vi "lockin - Set REF phase equals zero.vi"(9 "reset REF phi to zero":bool, 10 "Channels: Lockin":T1={"REF f (Hz)"=[0.4, 0.4], "REF phi (deg)"=[0.0, 0.0]} {"REF phi (deg)" format="%#_3g"}, 11 "Channels: AO":T2={"AO amp (V)"=[0.0, 0.0, 0.0, 0.0, 0.0, 0.0, 0.0, 0.0], "AO DC (V)"=[0.0, 0.0, 0.0, 0.0, 0.0, 0.0, 0.0, 0.0], "AO f (Hz)"=[0.4, 0.4, 0.4, 0.4, 0.4, 0.4, 0.4, 0.4], "AO phi (deg)"=[0.0, 0.0, 0.0, 0.0, 0.0, 0.0, 0.0, 0.0], "function"=[enum."Triangle Wave", enum."Sine Wave", enum."Sine Wave", enum."Sine Wave", enum."Sine Wave", enum."Sine Wave", enum."Sine Wave", enum."Sine Wave"]} {"AO f (Hz)" min=0.001 max=1000.0; "AO DC (V)" format="%#_6p"; "AO amp (V)" format="%#_6p"}) -> (2 "Channels: Lockin 2":T1, 3 "Channels: AO 2":T2)   [LabVIEW 2013]
panel:
  # "0"
  # "1"
  # "2"
  # "3"
  # "4"
  # "5"
  # "6"
  # "7"
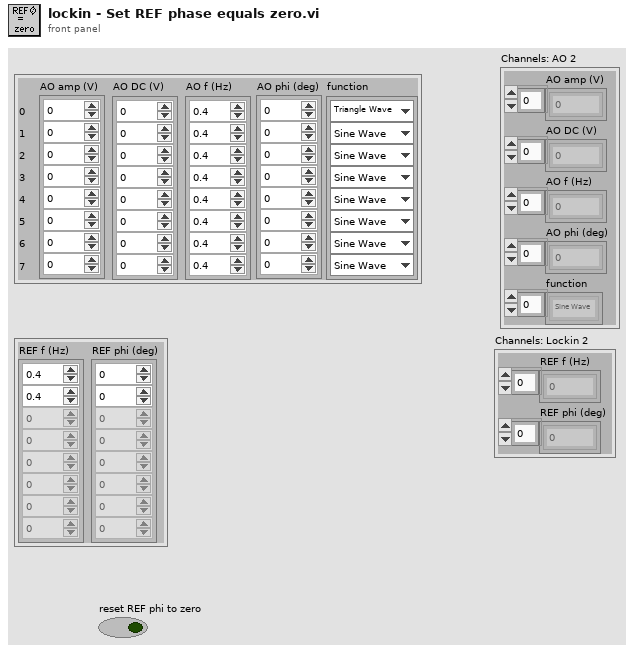
[diagram p1: front panel]
types:
  T1 = cluster{"REF f (Hz)":dbl[], "REF phi (deg)":dbl[]}
  T2 = cluster{"AO amp (V)":dbl[], "AO DC (V)":dbl[], "AO f (Hz)":dbl[], "AO phi (deg)":dbl[], "function":enum16{"Sine Wave", "Triangle Wave", "Square Wave", "Sawtooth Wave"}[]}
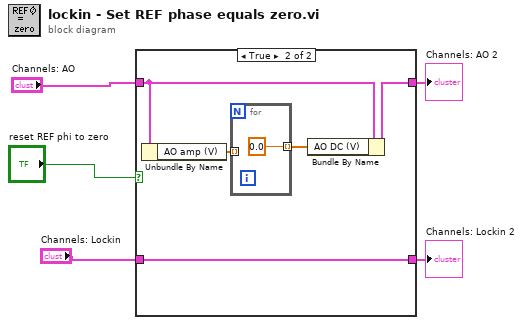
[diagram p0: block diagram]
diagram:
  n1 = case shown="True" "reset REF phi to zero" {
    tunnel: "Channels: AO" -> [w7 w10]
    tunnel: [w7 w12] -> w5
    tunnel: "Channels: Lockin" -> [w6 w11]
    tunnel: [w6 w11] -> w4
    frame False {
    }
    frame True {
      n2 = Unbundle By Name(w10) -> ("AO amp (V)"=w9:dbl[])
      n3 = for {
        tunnel: w9 -> [_] mode=indexing
        tunnel: [0.0] -> w8 mode=indexing
      }
      n4 = Bundle By Name(cluster=w10, "AO DC (V)"=w8) -> (w12:T2)
    }
  }
  "Channels: AO 2" <- w5
  "Channels: Lockin 2" <- w4
